vi "Global Enable Logging.vi"() -> ()   [LabVIEW 2020]
panel:
  in  "Enable Logging":bool
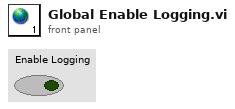
[diagram p1: front panel]
diagram:
